vi "再战使用Active与Excel的高速数据交互2014-10-14   2213 .vi"() -> ()   [LabVIEW 2014]
panel:
  out "用时：写入单元格数据":u32
  out "用时：打开指定Sheet":u32
  out "用时：打开指定Work":u32
  out "用时：总耗时":u32
  in  "要写入的数据8：完成时间":string
  in  "要写入的数据7：其他信息":string
  in  "要写入的数据1：追溯哈希值":string
  in  "初始放置的列":i32
  out "生成一个将要写入的数组":string[](array[string])
  in  "要写入的数据6：内圆同心度":string
  in  "要写入的数据5：外圆同心度":string
  in  "要写入的数据4：操作人员":string
  in  "要写入的数据3：追溯编号":string
  in  "要写入的数据2：图纸编号":string
  in  "输入参数三：错误输入":errorcluster
  in  "参数二：目标文件夹，就是被罗列的文件夹的路径":path
  in  "参数一：这里面放置被复制的模板文件":path
  in  "Excel._Worksheet":refnum<k7>
  in  "Excel._Application":refnum<k7>
  in  "Visible Boolean":bool=TRUE caption="按钮：文档是否可见"
  # "程序概述：\n目的：写入到EXCEl文档\n第一步：获取指定文件内的  文件和文件夹的  生成两个 字符串数组。这一步由LABVIEW 自带的VI完成\n第二步：判断EXCEL格式的文件中有没有以IMS生产数据记录+年+当前星期命名的文件，如果没有就新建，\n如果有就啥也不做。\n第三步：打开当前星期对应的EXCEL文件\n第四步：查看当前工作薄里面的SHEET文件里有没当前星期号命名的（比如当前是星期一 就看看有没有星期一）\n如果没有就新建 ，如果就啥事也不做。\n第五步：初始化赋值第一行数据，比如 图纸编号  同心度数据。。\n第六步：判断最小不为空的行号\n第七步：将指定数据写入进去\n第八步：关闭保存。\n至此结束IMS项目的数据保存任务。\nQQ：470885756  \nE-mail：wenluderen@gmail.com"
  # "第一步：获取指定文件内的  文件和文件夹的  生成两个 字符串数组。这一步由LABVIEW 自带的VI完成"
  # "目前的程序已经实现的数据的写入"
  # "第一步：打开并且显示"
  # "第四步：设定目标单元格值"
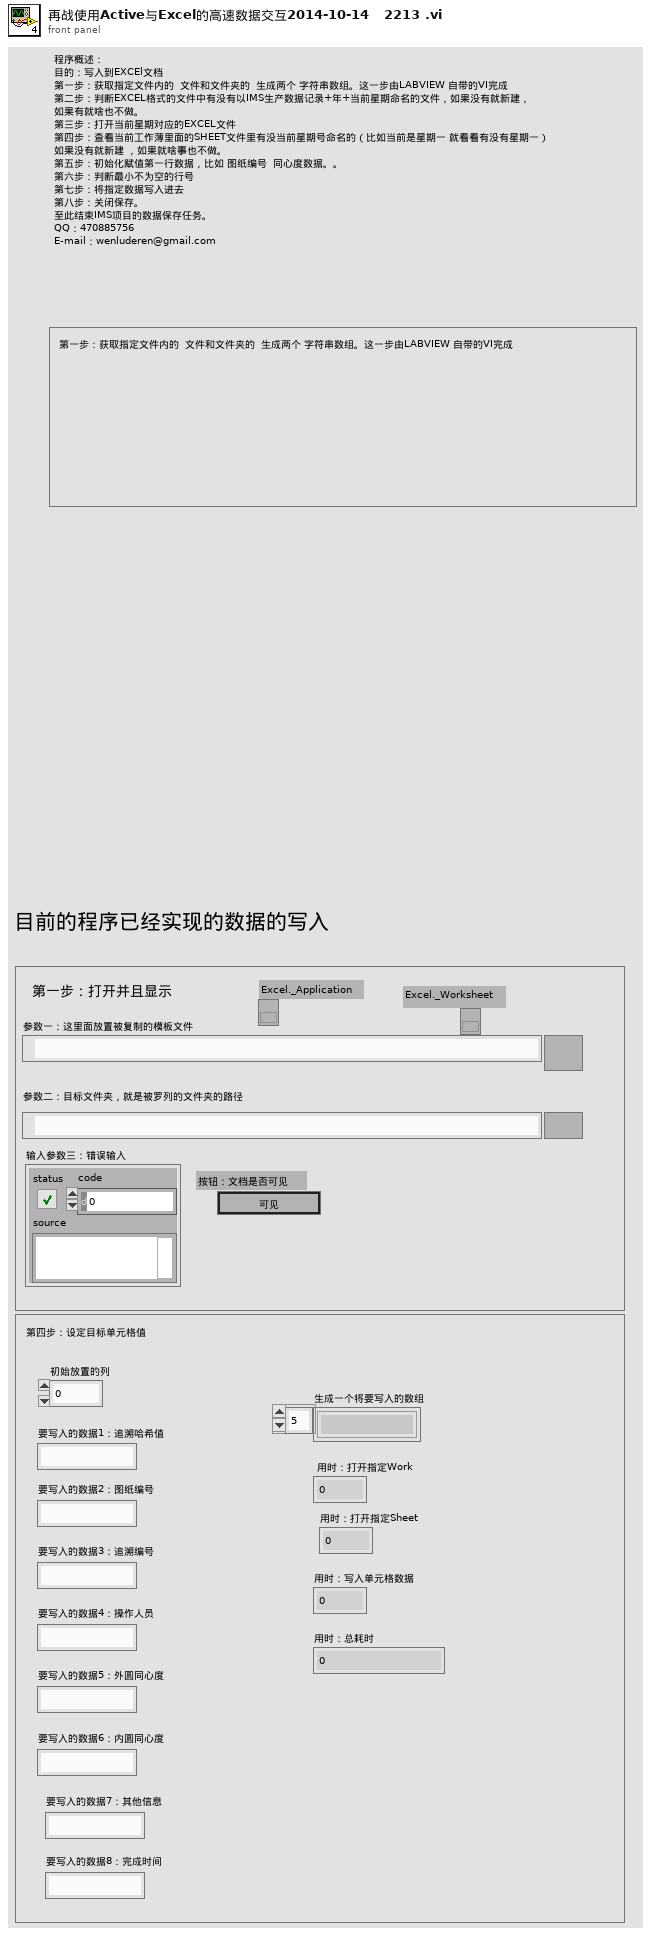
[diagram p1: front panel]
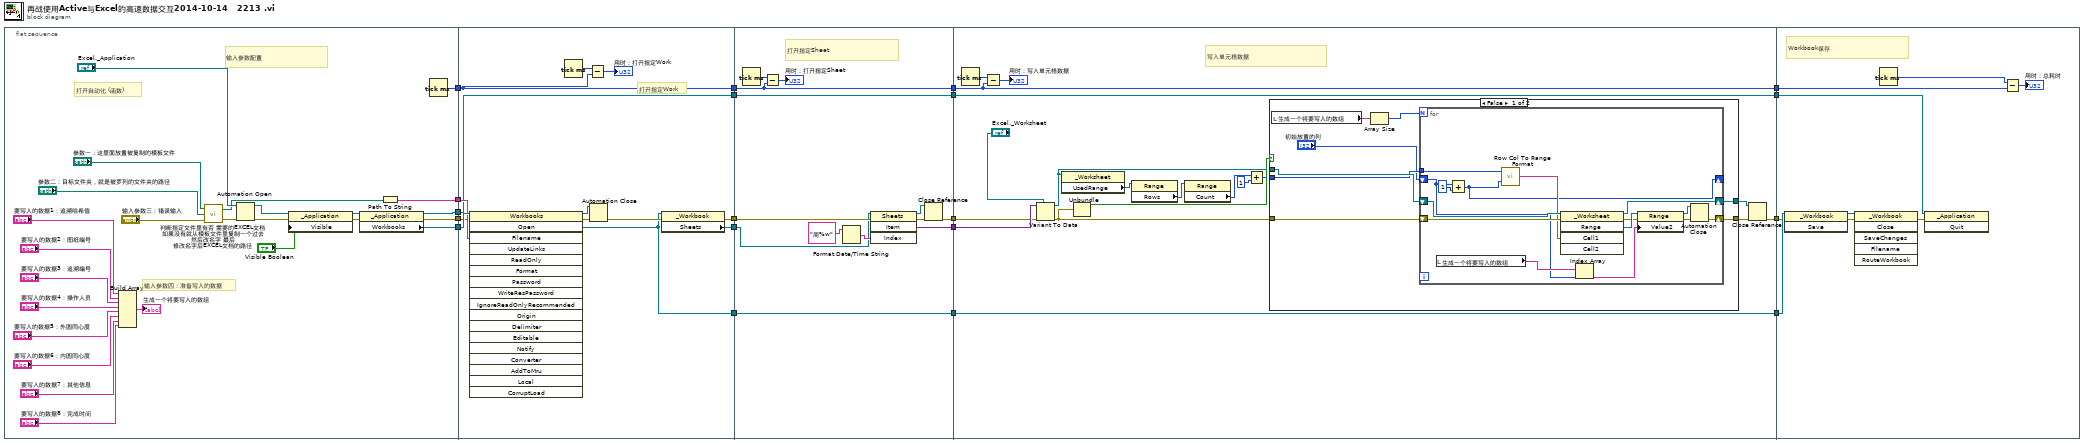
[diagram p0: block diagram]
diagram:
  n1 = flat-sequence {
    tunnel: [w38] -> w19
    tunnel: [w37] -> w18
    tunnel: [w36] -> w17
    tunnel: [w35] -> w5
    tunnel: [w25] -> w1
    tunnel: w19 -> [w54]
    tunnel: w18 -> [w53]
    tunnel: w17 -> [w52]
    tunnel: [w51] -> w15
    tunnel: [w50] -> w14
    tunnel: [w49] -> w10
    tunnel: [w48] -> w6
    tunnel: w5 -> [w48]
    tunnel: [w46] -> w2
    tunnel: w1 -> [w46]
    tunnel: [w67] -> w16
    tunnel: w15 -> [w61]
    tunnel: w14 -> [w68]
    tunnel: [w66] -> w13
    tunnel: [w63] -> w11
    tunnel: w10 -> [w63]
    tunnel: [w62] -> w7
    tunnel: w6 -> [w62]
    tunnel: [w59] -> w3
    tunnel: w2 -> [w59]
    tunnel: w16 -> [w87]
    tunnel: w13 -> [w83]
    tunnel: [w82] -> w12
    tunnel: w11 -> [w82]
    tunnel: [w81] -> w9
    tunnel: [w80] -> w8
    tunnel: w7 -> [w80]
    tunnel: [w72] -> w4
    tunnel: w3 -> [w72]
    tunnel: w12 -> [w123]
    tunnel: w9 -> [w122]
    tunnel: w8 -> [w118]
    tunnel: w4 -> [w115]
    frame #0 {
      # "输入参数四：准备写入的数据"
      # "输入参数配置"
      # "打开自动化 (函数)"
      n2 = Build Array("要写入的数据1：追溯哈希值", "要写入的数据2：图纸编号", "要写入的数据3：追溯编号", "要写入的数据4：操作人员", "要写入的数据5：外圆同心度", "要写入的数据6：内圆同心度", "要写入的数据7：其他信息", "要写入的数据8：完成时间") -> (→"生成一个将要写入的数组":string[])
      n3 = call "判断指定文件里有否 需要的EXCEL文档   如果没有就从模板文件里复制一个过去 然后改名字 最后  修改名字后EXCEL文档的路径.vi"("输入参数三：错误输入"="输入参数三：错误输入", "参数二：目标文件夹，就是被罗列的文件夹的路径"="参数二：目标文件夹，就是被罗列的文件夹的路径", "参数一：这里面放置被复制的模板文件"="参数一：这里面放置被复制的模板文件") -> ("输出参数二：错误输出"=w24:errorcluster, "输出参数一：修改完名字的路径"=w23:path)
      n4 = Automation Open(error in (no error)=w24, Automation Refnum="Excel._Application") -> (Automation Refnum=w43:refnum<k7>, error out=w44:errorcluster)  [unwired: 2 out]
      n5 = property class="_Application"(reference=w43, error in=w44, "Visible"="Visible Boolean") -> (reference out=w42:refnum<k7>, error out=w41:errorcluster)
      n6 = property class="_Application"(reference=w42, error in=w41) -> (reference out=w35:refnum<k7>, error out=w36:errorcluster, "Workbooks"=w38:refnum<k7>)
      n7 = Path To String(path=w23) -> (string=w37:string)
      n8 = Tick Count (ms)() -> (millisecond timer value=w25:u32)
    }
    frame #1 {
      # "打开指定Work"
      n9 = invoke class="Workbooks" method="Open"(reference=w54, error in=w52, "Filename"=w53) -> (reference out=w56:refnum<k7>, error out=w55:errorcluster, "Open"=w49:refnum<k7>)  [unwired: 15 in, 15 out]
      n10 = Tick Count (ms)() -> (millisecond timer value=w47:u32)
      n11 = Subtract(x=w47, y=w46) -> (x-y=→"用时：打开指定Work":u32)
      n12 = Automation Close(3:w55, 5:w56) -> (0:w57:errorcluster)
      n13 = property class="_Workbook"(reference=w49, error in=w57) -> (error out=w50:errorcluster, "Sheets"=w51:refnum<k7>)  [unwired: 1 out]
    }
    frame #2 {
      # "打开指定Sheet"
      n14 = Tick Count (ms)() -> (millisecond timer value=w60:u32)
      n15 = Subtract(x=w60, y=w59) -> (x-y=→"用时：打开指定Sheet":u32)
      n16 = Format Date/Time String(time format string (%c)="周%w") -> (date/time string=w69:string)  [unwired: 2 in]
      n17 = invoke class="Sheets" method="Item"(reference=w61, error in=w68, "Index"=w69) -> (reference out=w65:refnum<k7>, error out=w64:errorcluster, "Item"=w67:variant)  [unwired: 1 in, 1 out]
      n18 = Close Reference(reference=w65, error in (no error)=w64) -> (error out=w66:errorcluster)
    }
    frame #3 {
      # "写入单元格数据"
      n19 = Tick Count (ms)() -> (millisecond timer value=w73:u32)
      n20 = Subtract(x=w73, y=w72) -> (x-y=→"用时：写入单元格数据":u32)
      n21 = Variant To Data(error in=w83, type="Excel._Worksheet", Variant=w87) -> (data=w79:refnum<k7>, error out=w89:errorcluster)
      n22 = property class="_Worksheet"(reference=w79) -> ("UsedRange"=w78:refnum<k7>)  [unwired: 1 in, 2 out]
      n23 = Unbundle(w89) -> ("status"=w88:bool)  [unwired: 2 out]
      n24 = property class="Range"(reference=w78) -> ("Rows"=w77:refnum<k7>)  [unwired: 1 in, 2 out]
      n25 = property class="Range"(reference=w77) -> ("Count"=w74:i32)  [unwired: 1 in, 2 out]
      n26 = Add(x=w74, y=1) -> (x+y=w75:i32)
      n27 = case shown="False" w88 {
        tunnel: w89 -> [w94 w114]
        tunnel: [w97 w114] -> w86
        tunnel: [w96 w113] -> w85
        tunnel: w79 -> [w95 w113]
        tunnel: w75 -> [w93 _]
        frame False {
          n28 = local read "生成一个将要写入的数组"() -> (w90:string[])
          n29 = Array Size(array=w90) -> (size(s)=w92:i32)
          n30 = for {
            N: w92 -> [_]
            tunnel: w93 -> [w99]
            shift-right: [w107] -> w96
            shift-left: w95 -> [w106]
            shift-right: [w108] -> w97
            shift-left: w94 -> [w105]
            shift-right: [w98] -> _
            shift-left: "初始放置的列" -> [w101]
            n31 = local read "生成一个将要写入的数组"() -> (w102:string[])
            n32 = Add(x=w101, y=1) -> (x+y=w98:i32)
            n33 = call "Row Col To Range Format.vi"("Column"=w98, "Row"=w99) -> ("Output String"=w100:string)
            n34 = invoke class="_Worksheet" method="Range"(reference=w106, error in=w105, "Cell1"=w100) -> (reference out=w107:refnum<k7>, error out=w111:errorcluster, "Range"=w112:refnum<k7>)  [unwired: 2 in, 2 out]
            n35 = Index Array(array=w102, index=w101) -> (element=w103:string)
            n36 = property class="Range"(reference=w112, error in=w111, "Value2"=w103) -> (reference out=w110:refnum<k7>, error out=w109:errorcluster)
            n37 = Automation Close(3:w109, 5:w110) -> (0:w108:errorcluster)
          }
        }
        frame True {
        }
      }
      n38 = Close Reference(reference=w85, error in (no error)=w86) -> (error out=w81:errorcluster)
    }
    frame #4 {
      # "Workbook保存"
      n39 = invoke class="_Workbook" method="Save"(reference=w123, error in=w122) -> (reference out=w121:refnum<k7>, error out=w120:errorcluster)  [unwired: 1 in, 1 out]
      n40 = invoke class="_Workbook" method="Close"(reference=w121, error in=w120) -> (error out=w119:errorcluster)  [unwired: 4 in, 5 out]
      n41 = Tick Count (ms)() -> (millisecond timer value=w116:u32)
      n42 = invoke class="_Application" method="Quit"(reference=w118, error in=w119) -> ()  [unwired: 1 in, 3 out]
      n43 = Subtract(x=w116, y=w115) -> (x-y=→"用时：总耗时":u32)
    }
  }
